vi "4XNN.vi"(11 "Variables and Memory in":T1 {"GFX" format="%02x"}) -> (3 "Variables and Memory out":T1 {"GFX" format="%02x"})   [LabVIEW 2021]
uses:
  Controls/ClusterF.ctl
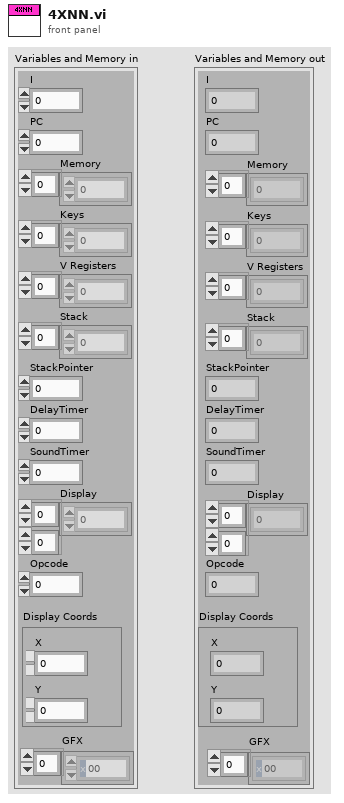
[diagram p1: front panel]
types:
  T1 = typedef "ClusterF.ctl" = cluster{"I":u16, "PC":u16, "Memory":u8[], "Keys":u8[], "V Registers":u8[], "Stack":u16[], "StackPointer":u16, "DelayTimer":u8, "SoundTimer":u8, "Display":u8[][], "Opcode":u16, "Display Coords":cluster{"X":u8, "Y":u8}, "GFX":u8[]}
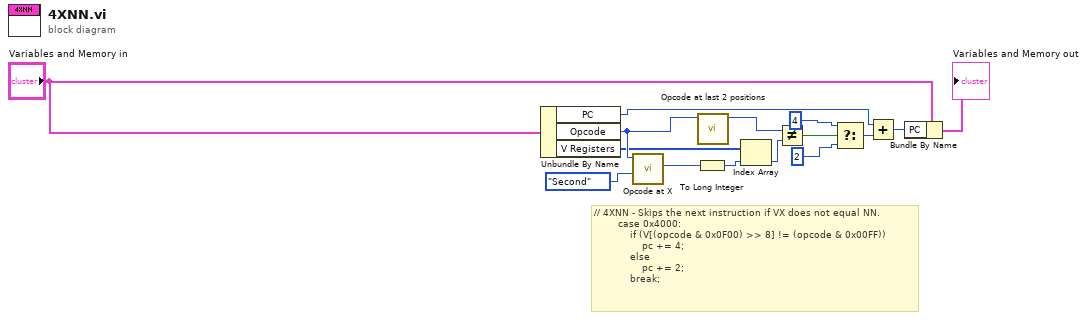
[diagram p0: block diagram]
diagram:
  # "// 4XNN - Skips the next instruction if VX does not equal NN.\n        case 0x4000:\n            if (V[(opcode & 0x0F00) >> 8] != (opcode & 0x00FF))\n                pc += 4;\n            else\n                pc += 2;\n            break;"
  n1 = Unbundle By Name("Variables and Memory in") -> ("PC"=w6:u16, "Opcode"=w8:u16, "V Registers"=w2:u8[])
  n2 = call "Opcode at X.vi"("X Position"=enum16{"First", "Second", "Third", "Fourth"}."Second", "Opcode"=w8) -> ("Opcode at X Position (U8)"=w3:u8)  [unwired: 9 in]
  n3 = To Long Integer(number=w3) -> (32bit integer=w9:i32)
  n4 = call "Opcode at last 2 positions.vi"("Opcode"=w8) -> ("00FF"=w5:u8)  [unwired: 10 in]
  n5 = Index Array(array=w2, index=w9) -> (element=w4:u8)
  n6 = Not Equal?(x=w5, y=w4) -> (x != y?=w14:bool)
  n7 = Select(t=u16 4 ("y"), s=w14, f=u16 2 ("y")) -> (s? t:f=w15:u16)
  n8 = Add(x=w6, y=w15) -> (x+y=w7:u16)
  n9 = Bundle By Name(cluster="Variables and Memory in", "PC"=w7) -> (→"Variables and Memory out":T1)
